vi "华为UPS2000-G-(1-3KVA)界面.vi"() -> ()   [LabVIEW 2016, in "环境动力监测库.lvlib" / "UPS库.lvlib"]
panel:
  out "Port":string
  out "IP":string
  out "x+1":u32
  in  "解除告警":bool
  out "通信":bool=TRUE
  out "串口":string
  in  "停止自检":bool
  in  "启动自检":bool
  out "UPS状态":T1
  out "电池状态":T2 {"电池状态" items=["休眠"=2, "浮充"=3, "均充"=4, "放电"=5]}
  out "UPS参数":T3 {"开机状态" items=["关机", "开机中", "开机失败", "开机完成"]}
  in  "查看型号":bool
  in  "重开串口":bool
  # "V"
  # "%"
  # "S"
  # "Ah"
  # "kVA"
  # "V"
  # "Hz"
  # "V"
  # "A"
  # "Hz"
  # "kW"
  # "kVA"
  # "%"
  # "℃"
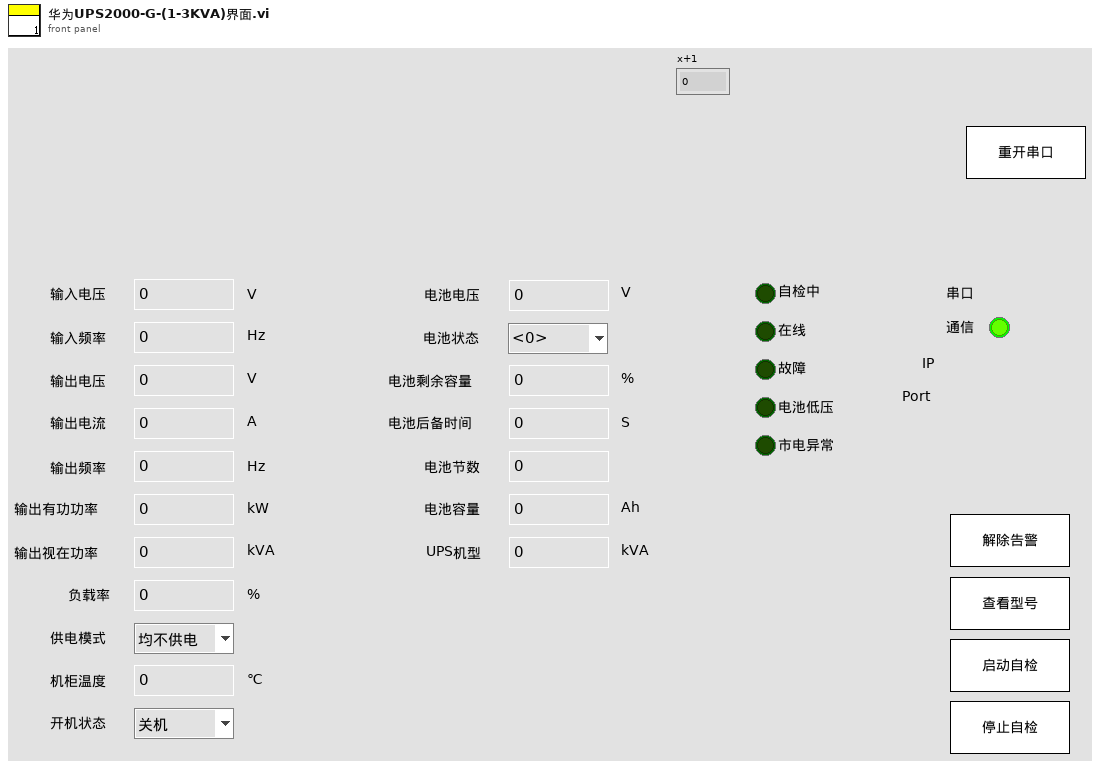
[diagram p1: front panel]
types:
  T1 = cluster{"保留":bool, "保留":bool, "自检中":bool, "在线":bool, "故障":bool, "保留":bool, "电池低压":bool, "市电异常":bool}
  T2 = cluster{"电池电压":dbl, "电池状态":u16, "电池剩余容量":u16, "电池后备时间":u32, "电池节数":u16, "电池容量":u16, "UPS机型":u16}
  T3 = cluster{"输入电压":dbl, "输入频率":dbl, "旁路电压V":dbl, "旁路频率HZ":dbl, "输出电压":dbl, "输出电流":dbl, "输出频率":dbl, "输出有功功率":dbl, "输出视在功率":dbl, "负载率":dbl, "供电模式":enum16{"均不供电", "旁路供电", "主路供电", "电池供电", "主路ECO"}, "输入制式0:单相":u16, "输出制式0:单相":u16, "机柜温度":dbl, "开机状态":u16, "UPS状态":u8}
  T4 = cluster{"VISA resource name":refnum<visa-resource-name>, "Serial Config":cluster{"baud rate (9600)":u32, "stop bits (10: 1 bit)":u16, "parity (0:none)":enum16{"None", "Odd", "Even", "Mark", "Space"}, "data bits (8)":u16, "timeout (10sec)":u32}, "型号选择":enum16{"山特UPSC1~3", "山特UPSC6~20", "华为UPS2000-G-(1-3KVA)"}, "HW-UPS-2000 MB session":refnum<class "MB_Master.lvclass">, "连接方式":enum16{"串口", "TCP"}, "IP":string, "Port":string}
  T5 = cluster{"输入电压V":dbl, "输入频率HZ":dbl, "旁路电压V":dbl, "旁路频率HZ":dbl, "输出电压V":dbl, "输出电流A":dbl, "输出频率HZ":dbl, "输出有功功率kW":dbl, "输出视在功率kVA":dbl, "负载率%":dbl, "供电模式":enum16{"均不供电", "旁路供电", "主路供电", "电池供电", "主路ECO"}, "输入制式0:单相":u16, "输出制式0:单相":u16, "机柜温度℃":dbl, "开机状态":u16, "UPS状态":u8}
  T6 = cluster{"电池电压V":dbl, "电池状态":u16, "电池剩余容量%":u16, "电池后备时间s":u32, "电池节数":u16, "电池容量AH":u16, "UPS机型KVA":u16}
  T7 = cluster{"市电":cluster{"状态":bool, "电压:":u16, "电流：":dbl, "详情  ":bool}, "UPS":cluster{"状态":bool, "输入电压:":sgl, "输出电压:":sgl, "电池电量:":u8, "电量":u16, "详情  ":bool}, "蓄电池12V":cluster{"状态":bool, "电压:":sgl, "电流:":sgl, "电池电量:":u8, "电量":u16, "详情  ":bool}, "蓄电池24V":cluster{"状态":bool, "电压:":sgl, "电流:":sgl, "电池电量:":u8, "电量":u16, "详情  ":bool}}
  T8 = cluster{"华为2000-G-UPS状态[0]":bool, "华为2000-G-UPS状态[1]":bool, "华为2000-G-UPS状态[2]":bool, "华为2000-G-UPS状态[3]":bool, "华为2000-G-UPS状态[4]":bool, "华为2000-G-UPS状态[5]":bool, "华为2000-G-UPS状态[6]":bool, "华为2000-G-UPS状态[7]":bool}
  T9 = cluster{"漏水监测输出":cluster{"漏水监测告警":bool, "告警内容":string}, "门禁监测输出":cluster{"门禁监测告警":bool, "告警内容":string}, "门禁监测输出2":cluster{"门禁监测告警":bool, "告警内容":string}, "温湿度监测输出":cluster{"温湿度监测告警":bool, "告警内容":string}, "烟雾监测输出":cluster{"烟雾监测告警":bool, "告警内容":string}, "空调监测输出":cluster{"空调监测告警":bool, "告警内容":string}, "自动重合闸输出":cluster{"自动重合闸告警":bool, "告警内容":string}, "红外入侵输出":cluster{"红外入侵告警":bool, "告警内容":string}, "振动输出":cluster{"振动告警":bool, "告警内容":string}, "UPS输出":cluster{"UPS告警":bool, "告警内容":string}, "蓄电池输出":cluster{"蓄电池告警":bool, "告警内容":string}, "蓄电池输出2":cluster{"蓄电池告警":bool, "告警内容":string}, "GPS输出":cluster{"定位告警":bool, "告警内容":string}, "北斗输出":cluster{"定位告警":bool, "告警内容":string}, "气象输出":cluster{"气象告警":bool, "告警内容":string}}
  T10 = enum32{"Bad", "Idle", "Run top level", "Running"}
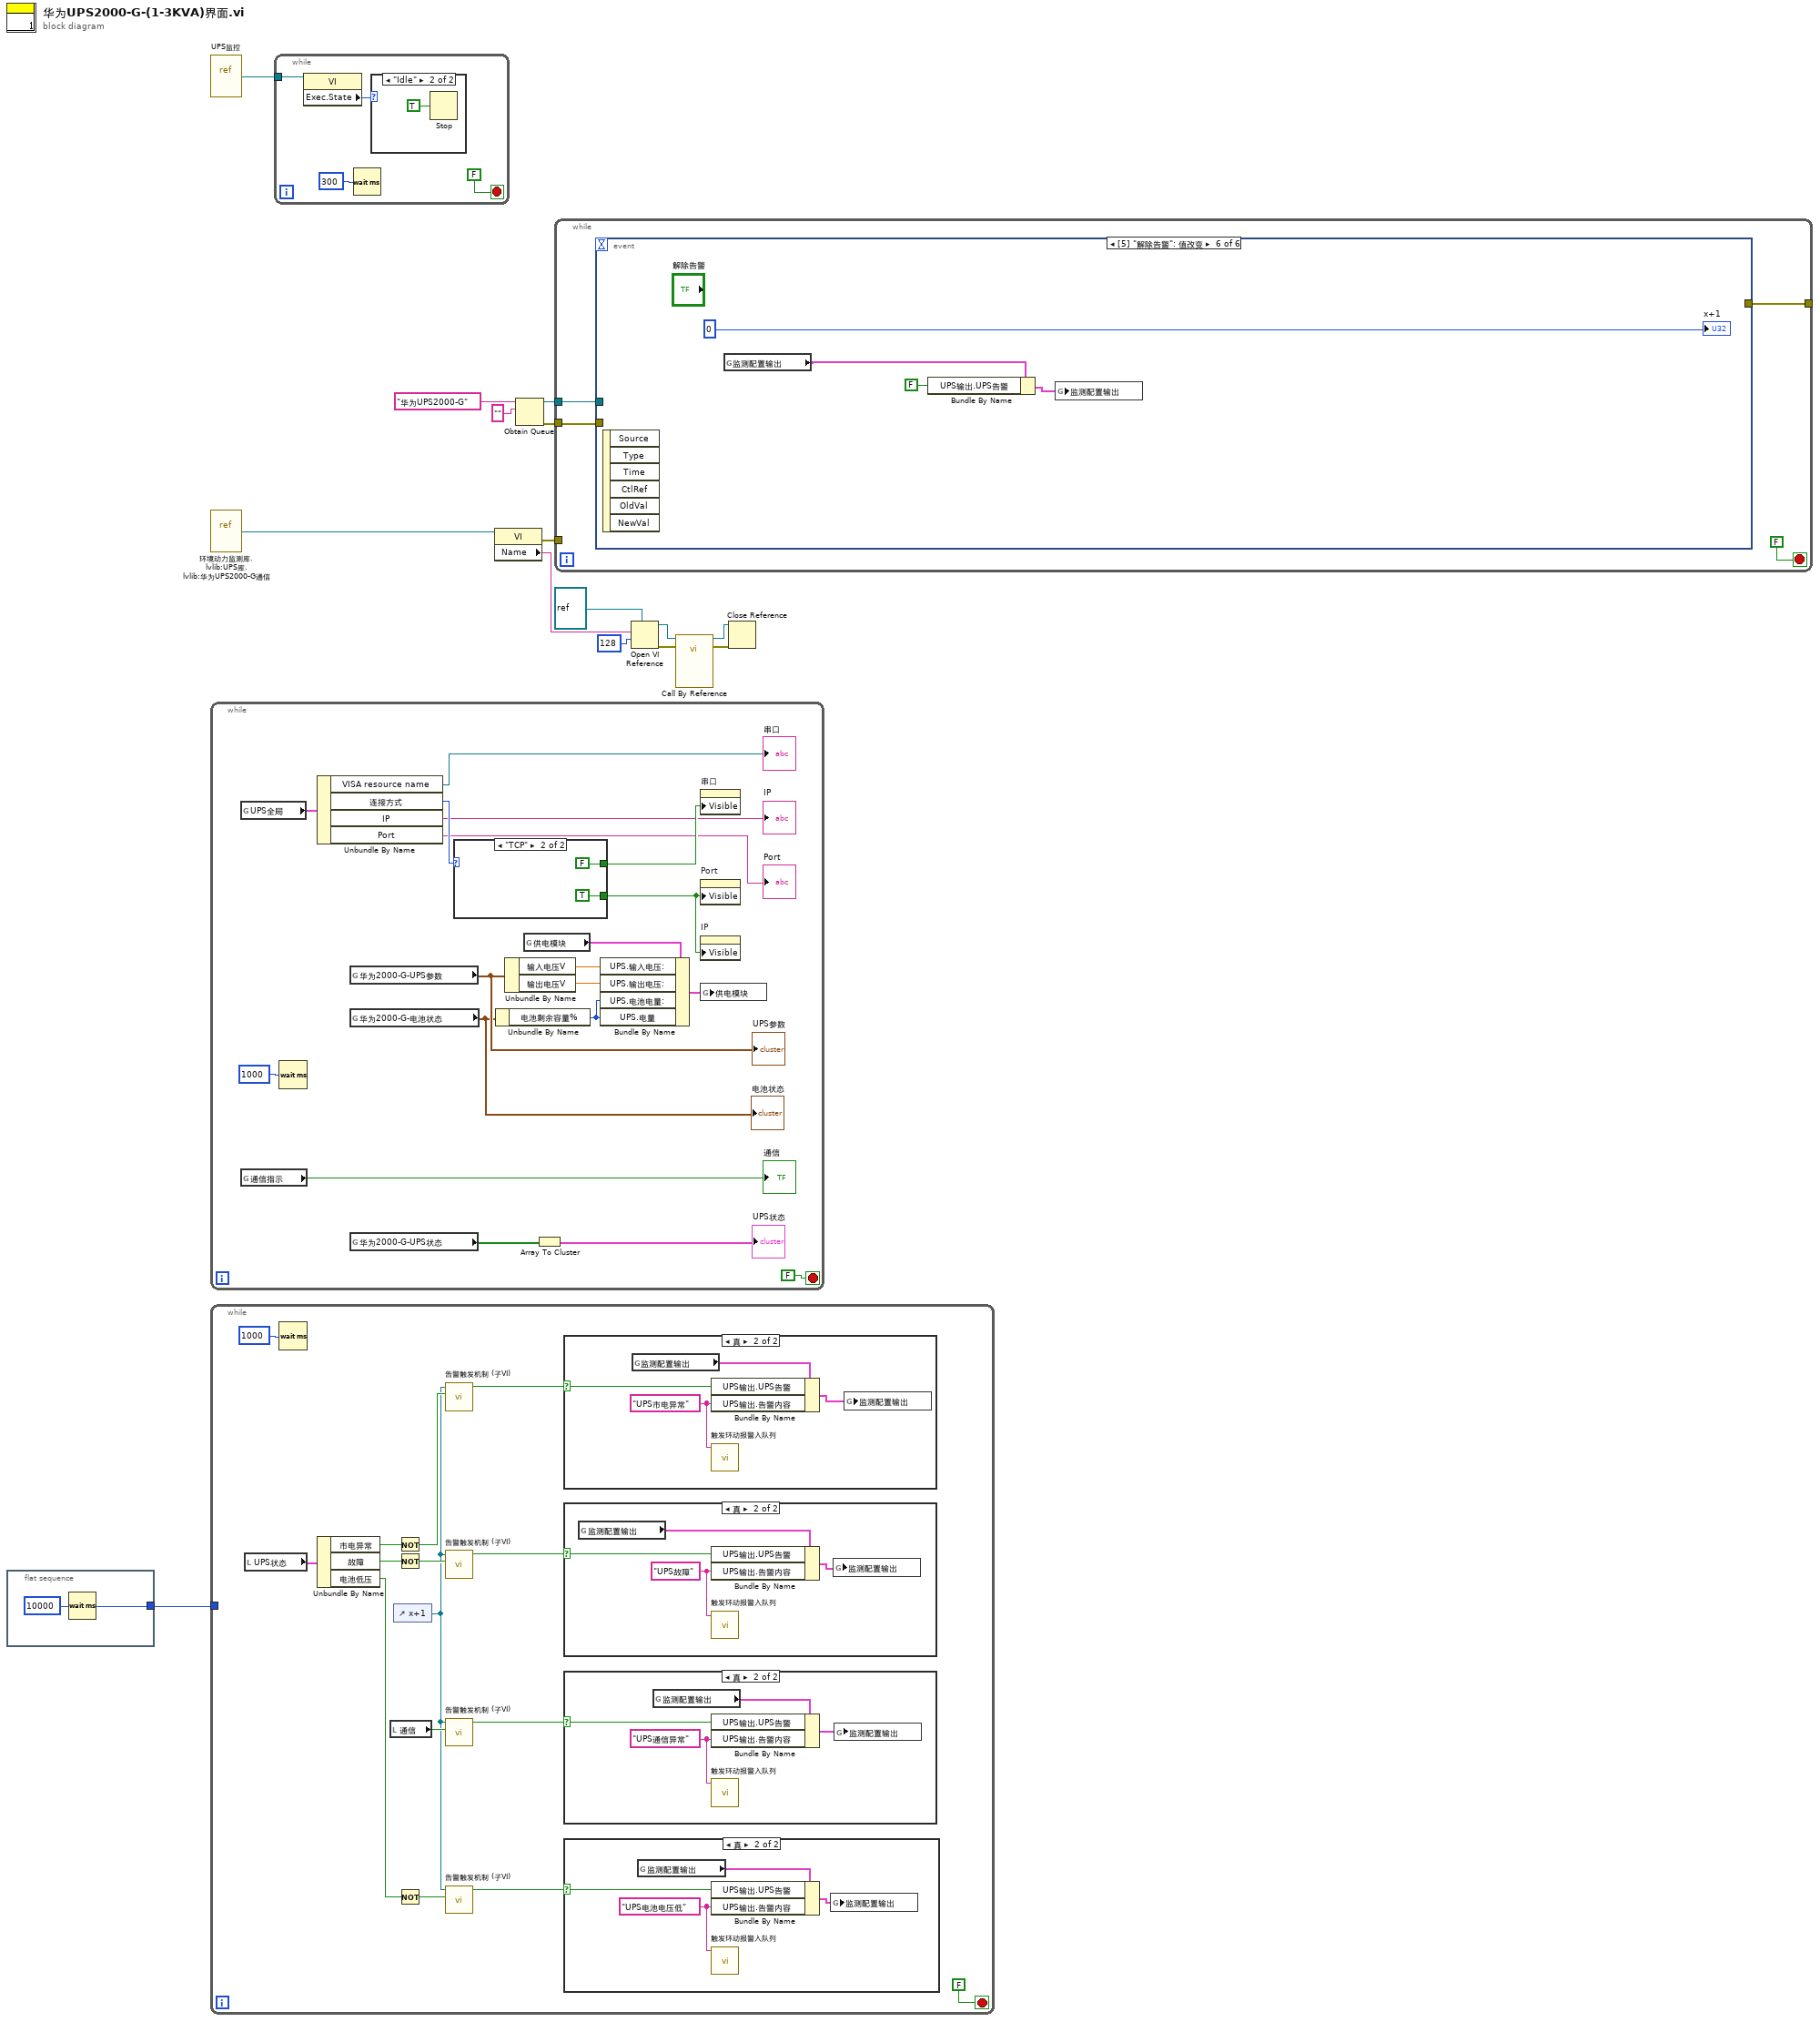
[diagram p0: block diagram]
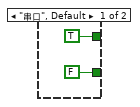
[diagram p7: hidden frame]
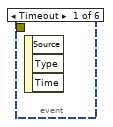
[diagram p8: hidden frame]
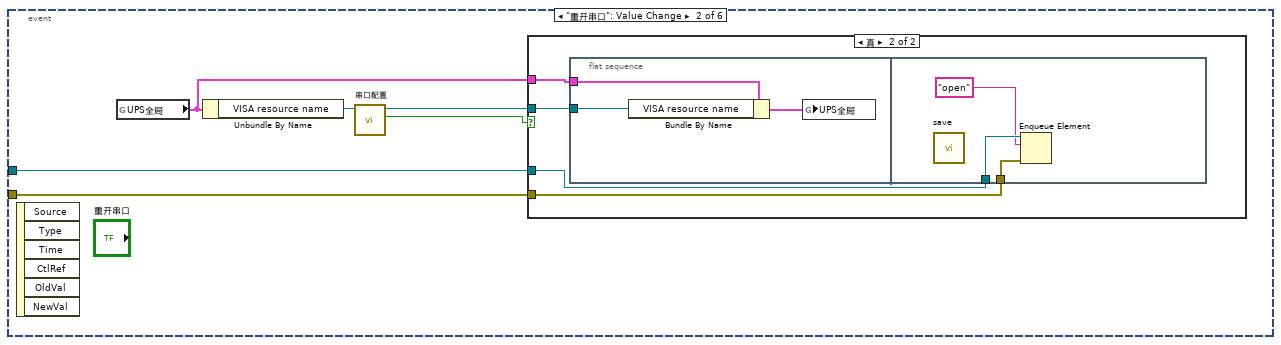
[diagram p9: hidden frame]
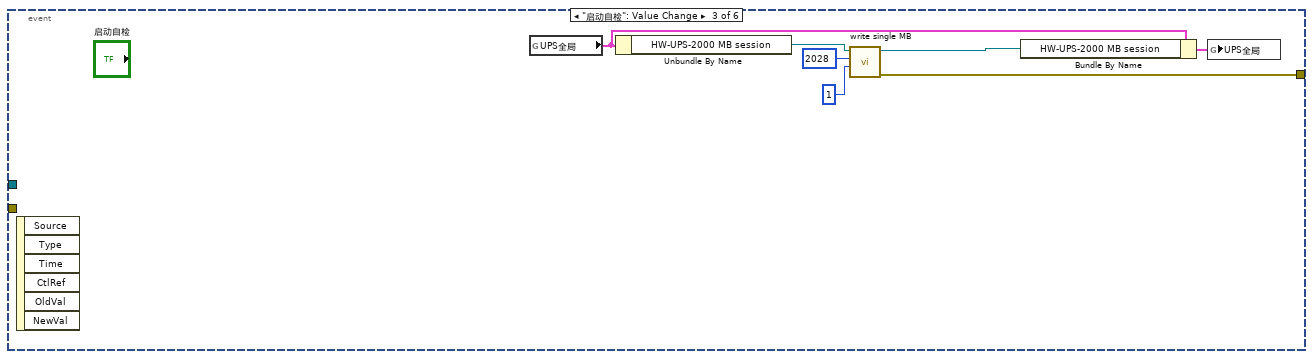
[diagram p11: hidden frame]
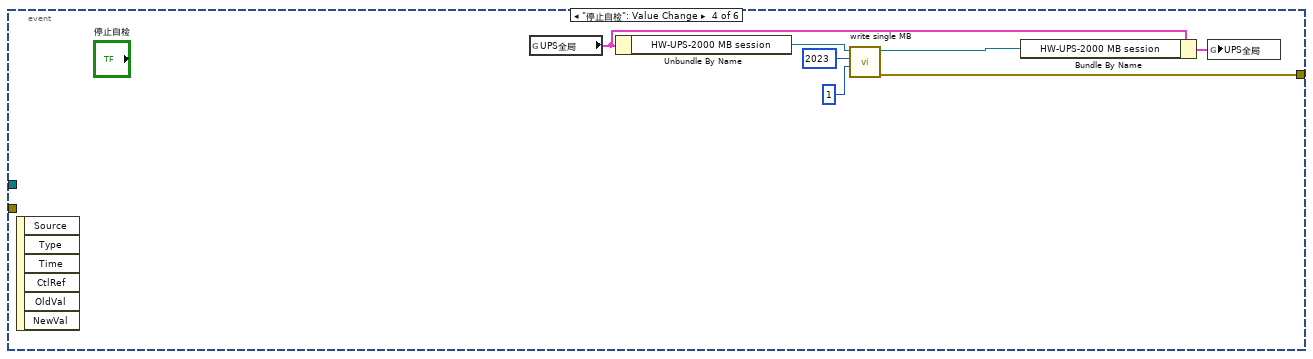
[diagram p12: hidden frame]
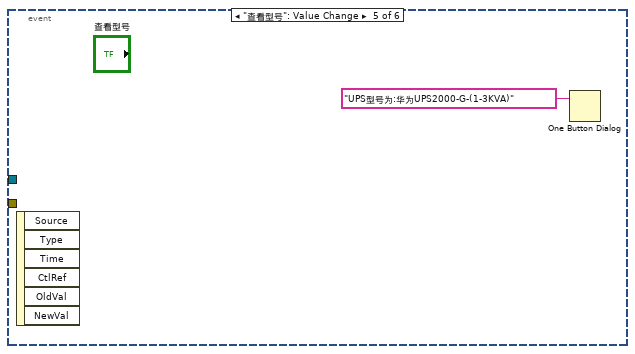
[diagram p13: hidden frame]
diagram:
  n1 = flat-sequence {
    tunnel: [w16] -> w1
    frame #0 {
      n2 = Wait (ms)(milliseconds to wait=u32 10000 ("等待时间（毫秒）")) -> (millisecond timer value=w16:u32)
    }
  }
  n3 = vi-ref "UPS监控.vi"() -> (w2:refnum<vi>)
  n4 = vi-ref "环境动力监测库.lvlib:UPS库.lvlib:华为UPS2000-G通信.vi"() -> (w8:refnum<vi>)
  n5 = while {
    stop <- FALSE stop-if-true
    n6 = global read "断电保存全局变量.vi" "UPS全局"() -> (w22:T4)
    n7 = global read "UPS内部交互全局.vi" "通信指示"() -> (→"通信":bool)
    n8 = Wait (ms)(milliseconds to wait=u32 1000 ("等待时间（毫秒）")) -> ()  [unwired: 1 out]
    n9 = Unbundle By Name(w22) -> ("VISA resource name"=→"串口":refnum<visa-resource-name>, "连接方式"=w20:enum16{"串口", "TCP"}, "IP"=→"IP":string, "Port"=→"Port":string)
    n10 = global read "UPS内部交互全局.vi" "华为2000-G-UPS参数"() -> (w31:T5)
    "UPS参数" <- w31
    n11 = global read "UPS内部交互全局.vi" "华为2000-G-电池状态"() -> (w28:T6)
    "电池状态" <- w28
    n12 = global read "UPS内部交互全局.vi" "华为2000-G-UPS状态"() -> (w26:bool[])
    n13 = case shown="\"TCP\"" w20 {
      tunnel: [TRUE FALSE] -> w24
      tunnel: [FALSE TRUE] -> w23
      frame "串口", Default {
      }
      frame "TCP" {
      }
    }
    n14 = Unbundle By Name(w28) -> ("电池剩余容量%"=w27:u16)
    n15 = Unbundle By Name(w31) -> ("输入电压V"=w30:dbl, "输出电压V"=w29:dbl)
    n16 = global read "内部交互全局变量.vi" "供电模块"() -> (w33:T7)
    n17 = Array To Cluster(array=w26) -> (cluster=→"UPS状态":T8)
    n18 = Bundle By Name(cluster=w33, "UPS.输入电压:"=w30, "UPS.输出电压:"=w29, "UPS.电池电量:"=w27, "UPS.电量"=w27) -> (w32:T7)
    n19 = property on="串口" class="Str"("Visible"=w24) -> ()  [unwired: 2 in, 2 out]
    n20 = property on="Port" class="Str"("Visible"=w23) -> ()  [unwired: 2 in, 2 out]
    n21 = property on="IP" class="Str"("Visible"=w23) -> ()  [unwired: 2 in, 2 out]
    n22 = global write "内部交互全局变量.vi" "供电模块"(w32) -> ()
  }
  n23 = while {
    tunnel: w1 -> [_]
    stop <- FALSE stop-if-true
    n24 = local read "UPS状态"() -> (w53:T1)
    n25 = Wait (ms)(milliseconds to wait=u32 1000 ("等待时间（毫秒）")) -> ()  [unwired: 1 out]
    n26 = Unbundle By Name(w53) -> ("市电异常"=w51:bool, "故障"=w48:bool, "电池低压"=w43:bool)
    n27 = local read "通信"() -> (w46:bool)
    n28 = control-ref of="x+1"() -> (w41:refnum<vi>)
    n29 = Not(x=w51) -> (.not. x?=w52:bool)
    n30 = Not(x=w48) -> (.not. x?=w49:bool)
    n31 = Not(x=w43) -> (.not. x?=w44:bool)
    n32 = call "告警触发机制 (子VI).vi"("状态输出"=w52, "Digital输入"=w41) -> ("触发告警"=w50:bool)  [unwired: 8 in, 1 out]
    n33 = call "告警触发机制 (子VI).vi"("状态输出"=w49, "Digital输入"=w41) -> ("触发告警"=w47:bool)  [unwired: 8 in, 1 out]
    n34 = call "告警触发机制 (子VI).vi"("状态输出"=w46, "Digital输入"=w41) -> ("触发告警"=w45:bool)  [unwired: 8 in, 1 out]
    n35 = call "告警触发机制 (子VI).vi"("状态输出"=w44, "Digital输入"=w41) -> ("触发告警"=w42:bool)  [unwired: 8 in, 1 out]
    n36 = case shown="真" w50 {
      selector: w50 -> [_ w70]
      frame False {
      }
      frame True {
        w71 = "UPS市电异常" ("报警内容")
        n37 = global read "内部交互全局变量.vi" "监测配置输出"() -> (w69:T9)
        n38 = Bundle By Name(cluster=w69, "UPS输出.UPS告警"=w70, "UPS输出.告警内容"=w71) -> (w68:T9)
        n39 = call "触发环动报警入队列.vi"("报警内容"=w71) -> ()  [unwired: 11 in]
        n40 = global write "内部交互全局变量.vi" "监测配置输出"(w68) -> ()
      }
    }
    n41 = case shown="真" w47 {
      selector: w47 -> [_ w58]
      frame False {
      }
      frame True {
        w59 = "UPS故障" ("报警内容")
        n42 = global read "内部交互全局变量.vi" "监测配置输出"() -> (w57:T9)
        n43 = Bundle By Name(cluster=w57, "UPS输出.UPS告警"=w58, "UPS输出.告警内容"=w59) -> (w56:T9)
        n44 = call "触发环动报警入队列.vi"("报警内容"=w59) -> ()  [unwired: 11 in]
        n45 = global write "内部交互全局变量.vi" "监测配置输出"(w56) -> ()
      }
    }
    n46 = case shown="真" w45 {
      selector: w45 -> [_ w62]
      frame False {
      }
      frame True {
        w63 = "UPS通信异常" ("报警内容")
        n47 = global read "内部交互全局变量.vi" "监测配置输出"() -> (w60:T9)
        n48 = Bundle By Name(cluster=w60, "UPS输出.UPS告警"=w62, "UPS输出.告警内容"=w63) -> (w61:T9)
        n49 = call "触发环动报警入队列.vi"("报警内容"=w63) -> ()  [unwired: 11 in]
        n50 = global write "内部交互全局变量.vi" "监测配置输出"(w61) -> ()
      }
    }
    n51 = case shown="真" w42 {
      selector: w42 -> [_ w66]
      frame False {
      }
      frame True {
        w67 = "UPS电池电压低" ("报警内容")
        n52 = global read "内部交互全局变量.vi" "监测配置输出"() -> (w65:T9)
        n53 = Bundle By Name(cluster=w65, "UPS输出.UPS告警"=w66, "UPS输出.告警内容"=w67) -> (w64:T9)
        n54 = call "触发环动报警入队列.vi"("报警内容"=w67) -> ()  [unwired: 11 in]
        n55 = global write "内部交互全局变量.vi" "监测配置输出"(w64) -> ()
      }
    }
  }
  n56 = while {
    tunnel: w2 -> [w75]
    stop <- FALSE stop-if-true
    n57 = property class="VI"(reference=w75) -> ("Exec.State"=w74:T10)  [unwired: 1 in, 2 out]
    n58 = Wait (ms)(milliseconds to wait=u32 300 ("等待时间（毫秒）")) -> ()  [unwired: 1 out]
    n59 = case shown="\"Idle\"" w74 {
      frame "Bad", Default {
      }
      frame "Idle" {
        n60 = Stop(stop? (T)=TRUE ("停止？(T)")) -> ()
      }
    }
  }
  n61 = property class="VI"(reference=w8) -> (error out=w4:errorcluster, "Name"=w9:string)  [unwired: 1 in, 1 out]
  n62 = Obtain Queue(name (unnamed)="华为UPS2000-G" ("名称（未命名）"), element data type="") -> (queue out=w6:refnum<queue>, error out=w5:errorcluster)  [unwired: 3 in, 1 out]
  n63 = while {
    tunnel: w5 -> [w79]
    tunnel: w6 -> [w78]
    tunnel: w4 -> [_]
    tunnel: [w77] -> _
    stop <- FALSE stop-if-true
    n64 = event shown="[5] \"解除告警\": 值改变" {
      selector: _ -> [_ _ _ _ _ _]
      dyn-events: _ -> [_ _ _ _ _ _]
      timeout: _ -> [_ _ _ _ _ _]
      tunnel: w79 -> [_ w83 _ _ _ _]
      tunnel: w78 -> [_ w84 _ _ _ _]
      tunnel: [_ _ w101 w108 _ _] -> w77
      event Timeout {
        n65 = event-data() -> ()  [unwired: 1 in, 3 out]
      }
      event "重开串口": Value Change {
        n66 = event-data() -> ()  [unwired: 1 in, 6 out]
        n67 = global read "断电保存全局变量.vi" "UPS全局"() -> (w81:T4)
        n68 = Unbundle By Name(w81) -> ("VISA resource name"=w82:refnum<visa-resource-name>)
        n69 = call "串口配置.vi"("请选择串口:"=w82) -> ("确认 2"=w86:bool, "请选择串口: 2"=w85:refnum<visa-resource-name>)  [unwired: 9 in]
        n70 = case shown="真" w86 {
          tunnel: w85 -> [_ w90]
          tunnel: w84 -> [_ w89]
          tunnel: w83 -> [_ w88]
          tunnel: w81 -> [_ w87]
          frame False {
          }
          frame True {
            n71 = flat-sequence {
              tunnel: w90 -> [w93]
              tunnel: w87 -> [w92]
              tunnel: w89 -> [w96]
              tunnel: w88 -> [w95]
              frame #0 {
                n72 = Bundle By Name(cluster=w92, "VISA resource name"=w93) -> (w91:T4)
                n73 = global write "断电保存全局变量.vi" "UPS全局"(w91) -> ()
              }
              frame #1 {
                n74 = call "save.vi"() -> ()  [unwired: 11 in, 1 out]
                n75 = Enqueue Element(queue=w96, element="open" ("元素"), error in (no error)=w95) -> ()  [unwired: 1 in, 3 out]
              }
            }
          }
        }
      }
      event "启动自检": Value Change {
        n76 = event-data() -> ()  [unwired: 1 in, 6 out]
        n77 = global read "断电保存全局变量.vi" "UPS全局"() -> (w97:T4)
        n78 = Unbundle By Name(w97) -> ("HW-UPS-2000 MB session"=w100:refnum<class "MB_Master.lvclass">)
        n79 = call "write single MB.vi"("value"=u16 1, "address"=u16 2028, "MB session in"=w100) -> ("error out"=w101:errorcluster, "MB session out"=w98:refnum<class "MB_Master.lvclass">)  [unwired: 7 in]
        n80 = Bundle By Name(cluster=w97, "HW-UPS-2000 MB session"=w98) -> (w99:T4)
        n81 = global write "断电保存全局变量.vi" "UPS全局"(w99) -> ()
      }
      event "停止自检": Value Change {
        n82 = event-data() -> ()  [unwired: 1 in, 6 out]
        n83 = global read "断电保存全局变量.vi" "UPS全局"() -> (w104:T4)
        n84 = Unbundle By Name(w104) -> ("HW-UPS-2000 MB session"=w107:refnum<class "MB_Master.lvclass">)
        n85 = call "write single MB.vi"("value"=u16 1, "address"=u16 2023, "MB session in"=w107) -> ("error out"=w108:errorcluster, "MB session out"=w105:refnum<class "MB_Master.lvclass">)  [unwired: 7 in]
        n86 = Bundle By Name(cluster=w104, "HW-UPS-2000 MB session"=w105) -> (w106:T4)
        n87 = global write "断电保存全局变量.vi" "UPS全局"(w106) -> ()
      }
      event "查看型号": Value Change {
        n88 = event-data() -> ()  [unwired: 1 in, 6 out]
        n89 = One Button Dialog(message="UPS型号为:华为UPS2000-G-(1-3KVA)" ("消息")) -> ()  [unwired: 1 in, 1 out]
      }
      event "解除告警": Value Change {
        n90 = event-data() -> ()  [unwired: 1 in, 6 out]
        n91 = global read "内部交互全局变量.vi" "监测配置输出"() -> (w113:T9)
        n92 = Bundle By Name(cluster=w113, "UPS输出.UPS告警"=FALSE) -> (w112:T9)
        n93 = global write "内部交互全局变量.vi" "监测配置输出"(w112) -> ()
        "x+1" <- u32 0 ("x+1")
      }
    }
  }
  n94 = Open VI Reference(type specifier VI Refnum (for type only)=refnum<vi> refnum, vi path=w9, options=128 ("选项")) -> (vi reference=w11:refnum<vi>, error out=w13:errorcluster)  [unwired: 3 in]
  n95 = call-by-ref "?"(reference=w11, error in=w13) -> (reference out=w15:refnum<vi>, error out=w14:errorcluster)  [unwired: 12 in]
  n96 = Close Reference(reference=w15, error in (no error)=w14) -> ()  [unwired: 1 out]
